vi "Read Name.vi"(8 "error in (no error)":errorcluster, 11 "Person in":refnum<class "Person.lvclass">) -> (0 "error out":errorcluster, 2 "Name":string, 3 "Person out":refnum<class "Person.lvclass">)   [LabVIEW 2023, in "Person.lvlib" / "Person.lvclass"]
doc: "Accessor method to read the Person's name."
uses:
  Person.lvclass
  Person.lvclass/Person.ctl
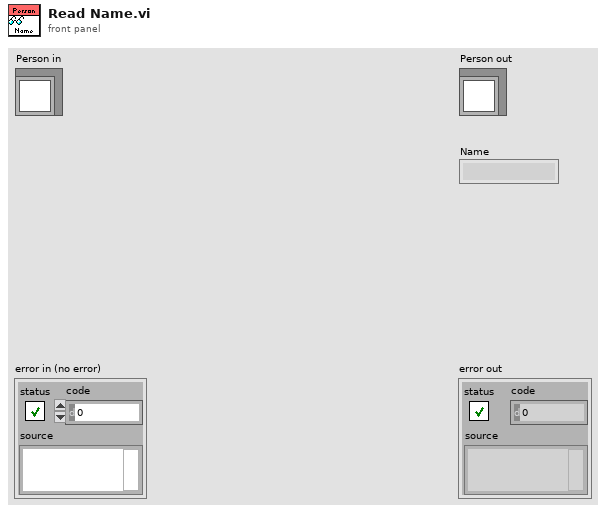
[diagram p1: front panel]
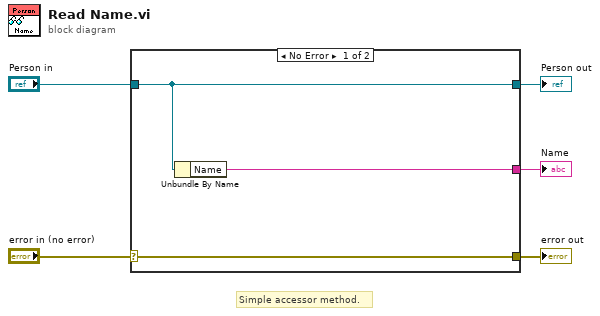
[diagram p0: block diagram]
diagram:
  # "Simple accessor method."
  n1 = case shown="No Error" "error in (no error)" {
    selector: "error in (no error)" -> [w8 w9]
    tunnel: [w8 w9] -> w4
    tunnel: [w7 w10] -> w2
    tunnel: "Person in" -> [w7 w10]
    tunnel: [w6 _] -> w1
    frame No Error {
      n2 = Unbundle By Name(w7) -> ("Name"=w6:string)
    }
    frame Error {
    }
  }
  "error out" <- w4
  "Person out" <- w2
  "Name" <- w1
